vi "ServiceHostReply.vi"(0 "Service ROS info in":T1={"topic port"=0, "Node"="", "topic"="", "type"="", "node port"=0, "error "={"status"=FALSE, "code"=0, "source"=""}, "Direction"=enum."Node", "Update (ms)"=1, "FIFO size"=1}, 2 "Reply":string) -> (1 "error out":errorcluster)   [LabVIEW 2012]
doc: "Replies to a Service Client (the service provider is started in the Service Host Wait). Do not use this VI without the Service Host Wait first."
uses:
  <userlib>/ROS for LabVIEW Software/ROS/Code/SubVIs/_ROSControl.ctl
  <userlib>/ROS for LabVIEW Software/ROS/Code/SubVIs/_ROSDirection.ctl
  <userlib>/ROS for LabVIEW Software/ROS/MessageBuilding/std_msgs/subs/stringScalar.vi
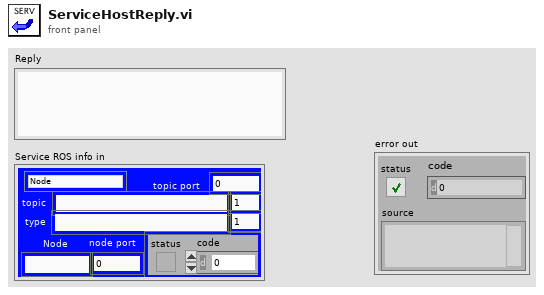
[diagram p1: front panel]
types:
  T1 = typedef "_ROSControl.ctl" = cluster{"topic port":u16, "Node":string, "topic":string, "type":string, "node port":u16, "error ":errorcluster, "Direction":T2, "Update (ms)":u16, "FIFO size":u16}
  T2 = typedef "_ROSDirection.ctl" = enum16{"Node", "Publisher", "Subscriber", "ServiceClient", "ServiceProvider"}
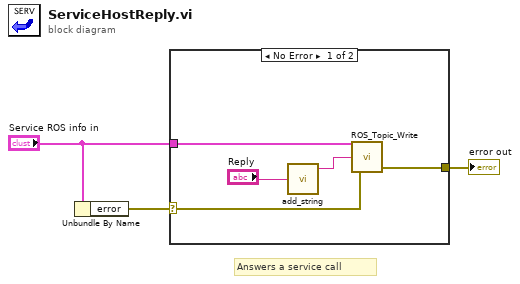
[diagram p0: block diagram]
diagram:
  # "Answers a service call"
  n1 = Unbundle By Name("Service ROS info in") -> ("error"=w1:errorcluster)
  n2 = case shown="No Error" w1 {
    selector: w1 -> [w5 w9]
    tunnel: "Service ROS info in" -> [w6 _]
    tunnel: [w8 w9] -> w3
    frame No Error {
      n3 = call-poly <userlib>:"add_string.vi"("String"="Reply") -> ("msg out"=w7:string)  [unwired: 4 in]
      n4 = call <userlib>:"ROS_Topic_Write.vi"("error in (no error)"=w5, "Msg in"=w7, "ROS in"=w6) -> ("error out"=w8:errorcluster)  [unwired: 1 in, 1 out]
    }
    frame Error {
    }
  }
  "error out" <- w3
